vi "Settings UI.vi"(8 "error in (no error)":errorcluster) -> (0 "error out":errorcluster)   [LabVIEW 2018]
uses:
  aef4f24d-ab5d-45ce-b2b0-1c0f110d7c04.vi
  be261c10-cb5d-4756-9ef8-d232eca7f9fa.vi
  bcb6971a-7736-4d1c-8bfd-29f94ac8081e.vi
  ec5355e7-4708-480d-bb95-c7978adf3668.vi
  <vilib>/JDP Science/JSONtext/String Subset.vi
  Wizard Config/Wizard Strings.vi
  <vilib>/JDP Science/JSONtext/Parsing/Parse Full Path or Item Name.vi
  <vilib>/JDP Science/JSONtext/Offset/Find Item Locations by Path.vi
  <vilib>/JDP Science/JSONtext/JSON text to Variant.vi
  <vilib>/JDP Science/JSONtext/Variant to JSON Text.vi
  <vilib>/JDP Science/JSONtext/JSONtext.lvlib
panel:
  in  "Include Evaluation String Comment":bool
  in  "Conditional Disable Structure Placement":string(combo)
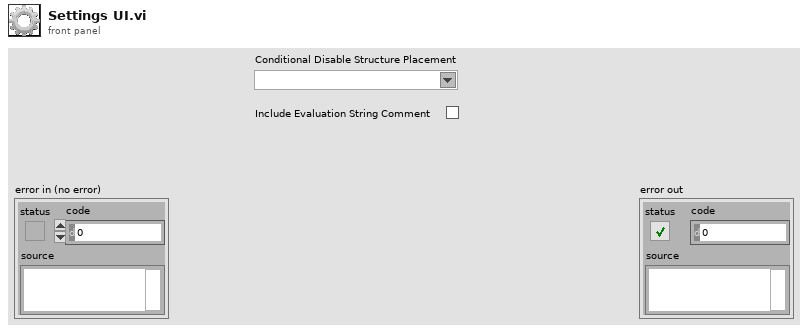
[diagram p1: front panel]
types:
  T1 = enum32{"Invalid", "Standard", "Closed", "Hidden", "Minimized", "Maximized"}
  T2 = enum16{"open", "replace", "create", "open or create", "replace or create", "replace or create with confirmation"}
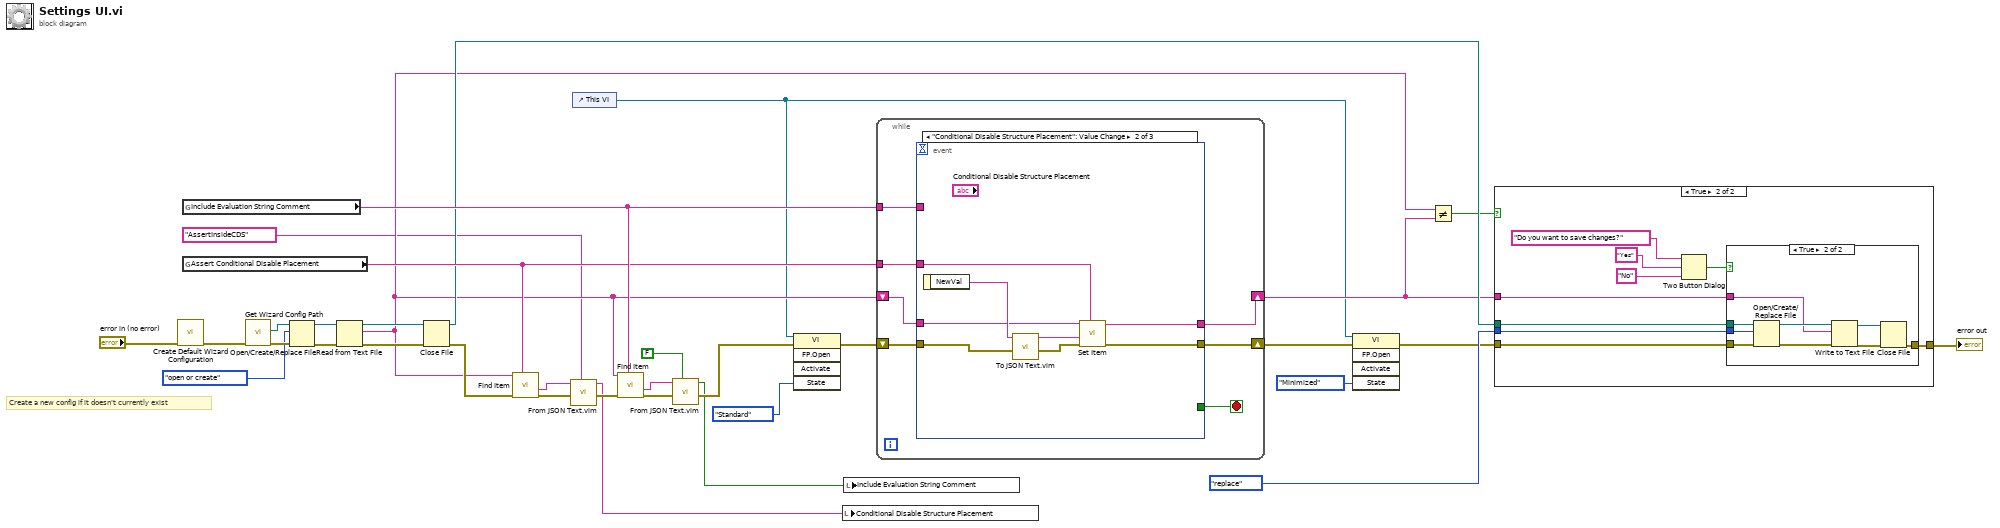
[diagram p0: block diagram]
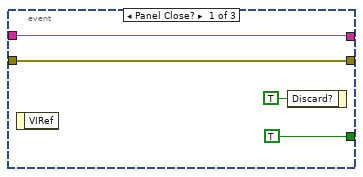
[diagram p4: hidden frame]
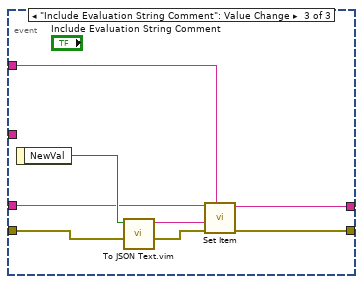
[diagram p5: hidden frame]
diagram:
  # "Create a new config if it doesn't currently exist"
  n1 = call "Create Default Wizard Configuration.vi"("error in (no error)"="error in (no error)") -> ("error out"=w21:errorcluster)  [unwired: 9 in, 1 out]
  n2 = global read "Wizard Strings.vi" "Include Evaluation String Comment"() -> (w23:string)
  n3 = global read "Wizard Strings.vi" "Assert Conditional Disable Placement"() -> (w22:string)
  n4 = call "Get Wizard Config Path.vi"("error in (no error)"=w21) -> ("error out"=w20:errorcluster, "Wizard Config Path"=w19:path)  [unwired: 8 in, 1 out]
  n5 = Open/Create/Replace File(file path (use dialog)=w19, error in=w20, operation (0:open)=T2."open or create") -> (refnum out=w16:refnum<file>, error out=w17:errorcluster)  [unwired: 3 in, 1 out]
  n6 = Read from Text File(file (use dialog)=w16, error in=w17) -> (refnum out=w14:refnum<file>, text=w10:string, error out=w33:errorcluster)  [unwired: 2 in, 1 out]
  n7 = Close File(refnum=w14, error in=w33) -> (path=w13:path, error out=w15:errorcluster)
  n8 = call <vilib>:"Find Item.vi"("$Path or Item Name"=w22, "error in (no error)"=w15, "JSON"=w10) -> ("error out"=w32:errorcluster, "<JSON>"=w31:string)  [unwired: 5 in, 2 out]
  n9 = call "From JSON Text.vim"("Data Type and Default Value"="AssertInsideCDS" ("Conditional Disable Structure Placement"), "error in (no error)"=w32, "JSON"=w31) -> ("error out"=w30:errorcluster, "Data out"=w24:string)  [unwired: 7 in]
  n10 = control-ref of="This VI"() -> (w3:refnum<vi>)
  n11 = call <vilib>:"Find Item.vi"("$Path or Item Name"=w23, "error in (no error)"=w30, "JSON"=w10) -> ("error out"=w29:errorcluster, "<JSON>"=w28:string)  [unwired: 5 in, 2 out]
  n12 = call "From JSON Text.vim"("Data Type and Default Value"=FALSE, "error in (no error)"=w29, "JSON"=w28) -> ("error out"=w26:errorcluster, "Data out"=w25:bool)  [unwired: 7 in]
  n13 = invoke class="VI" method="FP.Open"(reference=w3, error in=w26, "State"=T1."Standard") -> (error out=w5:errorcluster)  [unwired: 2 in, 4 out]
  n14 = local write "Conditional Disable Structure Placement"(w24) -> ()
  n15 = local write "Include Evaluation String Comment"(w25) -> ()
  n16 = while {
    shift-right: [w37] -> w11
    shift-left: w10 -> [w38]
    shift-right: [w41] -> w34
    shift-left: w5 -> [w39]
    tunnel: w23 -> [w36]
    tunnel: w22 -> [w35]
    stop <- w40 stop-if-true
    n17 = event shown="[1] \"Conditional Disable Structure Placement\": Value Change" {
      selector: _ -> [_ _ _]
      dyn-events: _ -> [_ _ _]
      timeout: _ -> [_ _ _]
      tunnel: [w44 w47 w55] -> w41
      tunnel: w39 -> [w44 w53 w61]
      tunnel: [TRUE ("Discard?") _ _] -> w40
      tunnel: w38 -> [w42 w49 w57]
      tunnel: [w42 w48 w56] -> w37
      tunnel: w36 -> [_ _ w54]
      tunnel: w35 -> [_ w46 _]
      event Panel Close? {
        n18 = event-data() -> ()  [unwired: 1 in, 1 out]
        n19 = event-data("Discard?"=TRUE) -> ()  [unwired: 1 in, 1 out]
      }
      event "Conditional Disable Structure Placement": Value Change {
        n20 = event-data() -> ("NewVal"=w52:string)  [unwired: 1 in]
        n21 = call "To JSON Text.vim"("error in (no error)"=w53, "Anything"=w52) -> ("error out"=w51:errorcluster, "<JSON>"=w50:string)  [unwired: 8 in]
        n22 = call <vilib>:"Set Item.vi"("$Path or Item Name"=w46, "error in (no error)"=w51, "JSON to Insert"=w50, "JSON"=w49) -> ("error out"=w47:errorcluster, "<JSON>"=w48:string)  [unwired: 4 in, 1 out]
      }
      event "Include Evaluation String Comment": Value Change {
        n23 = event-data() -> ("NewVal"=w60:bool)  [unwired: 1 in]
        n24 = call "To JSON Text.vim"("error in (no error)"=w61, "Anything"=w60) -> ("error out"=w59:errorcluster, "<JSON>"=w58:string)  [unwired: 8 in]
        n25 = call <vilib>:"Set Item.vi"("$Path or Item Name"=w54, "error in (no error)"=w59, "JSON to Insert"=w58, "JSON"=w57) -> ("error out"=w55:errorcluster, "<JSON>"=w56:string)  [unwired: 4 in, 1 out]
      }
    }
  }
  n26 = invoke class="VI" method="FP.Open"(reference=w3, error in=w34, "State"=T1."Minimized") -> (error out=w4:errorcluster)  [unwired: 2 in, 4 out]
  n27 = Not Equal?(x=w10, y=w11) -> (x != y?=w8:bool)
  n28 = case shown="True" w8 {
    tunnel: w4 -> [w62 w71]
    tunnel: w13 -> [_ w70]
    tunnel: T2."replace" ("operation (0:open)") -> [_ w69]
    tunnel: w11 -> [_ w68]
    tunnel: [w62 w67] -> w9
    frame False {
    }
    frame True {
      n29 = Two Button Dialog(message="Do you want to save changes?", 1:"No" ("F button name (\"Cancel\")"), 2:"Yes" ("T button name (\"OK\")")) -> (T button?=w63:bool)
      n30 = case shown="True" w63 {
        tunnel: w71 -> [w72 w81]
        tunnel: w70 -> [_ w77]
        tunnel: w69 -> [_ w75]
        tunnel: w68 -> [_ w74]
        tunnel: [w72 w73] -> w67
        frame False {
        }
        frame True {
          n31 = Open/Create/Replace File(file path (use dialog)=w77, error in=w81, operation (0:open)=w75) -> (refnum out=w76:refnum<file>, error out=w78:errorcluster)  [unwired: 3 in, 1 out]
          n32 = Write to Text File(file (use dialog)=w76, text=w74, error in=w78) -> (refnum out=w80:refnum<file>, error out=w79:errorcluster)  [unwired: 1 in, 1 out]
          n33 = Close File(refnum=w80, error in=w79) -> (error out=w73:errorcluster)  [unwired: 1 out]
        }
      }
    }
  }
  "error out" <- w9
